vi "test_color_box.vi"() -> ()   [LabVIEW 2016]
panel:
  out "Boolean 3":bool
  in  "Color Box":u32(colorbox)
  in  "Boolean 2":bool
  out "Colors [4]":cluster{u32, u32}[](array[cluster])
  out "Boolean":bool
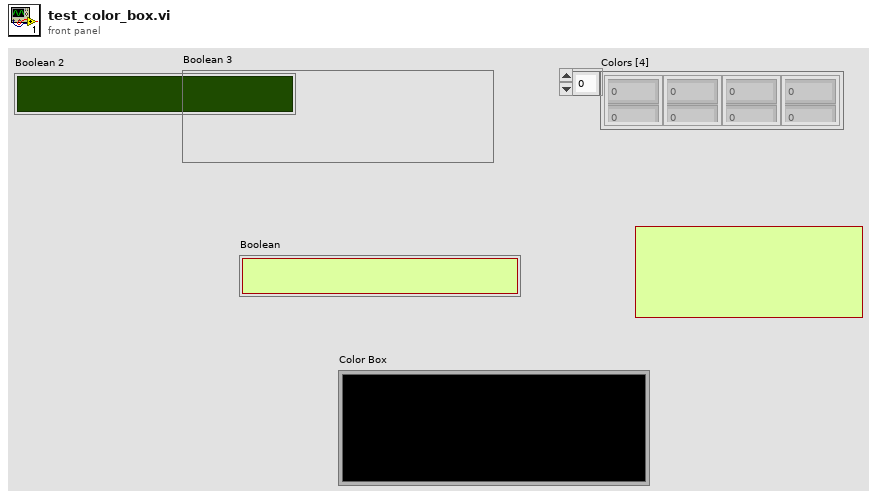
[diagram p1: front panel]
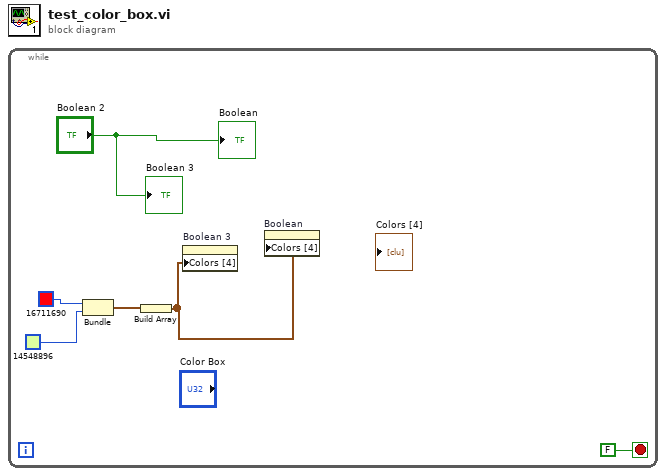
[diagram p0: block diagram]
diagram:
  n1 = while {
    stop <- FALSE stop-if-true
    n2 = Bundle(u32 16711690, u32 14548896) -> (w4:cluster{u32, u32})  [unwired: 1 in]
    n3 = Build Array(w4) -> (w3:cluster{u32, u32}[])
    n4 = property on="Boolean 3" class="Bool (strict)"("Colors [4]"=w3) -> ()  [unwired: 2 in, 2 out]
    n5 = property on="Boolean" class="Bool (strict)"("Colors [4]"=w3) -> ()  [unwired: 2 in, 2 out]
    "Boolean" <- "Boolean 2"
    "Boolean 3" <- "Boolean 2"
  }
